vi "Get_Mean_Path_Velocities-1.vi"(4 "error IN":errorcluster, 7 "[IN] Tracks + Starting Position":cluster{"Tracks":dbl[], "Start Pos":i32}[](array[cluster])) -> (0 "error OUT":errorcluster, 3 "[OUT] Mean Path Velocities":dbl[](array[numeric]))   [LabVIEW 2013]
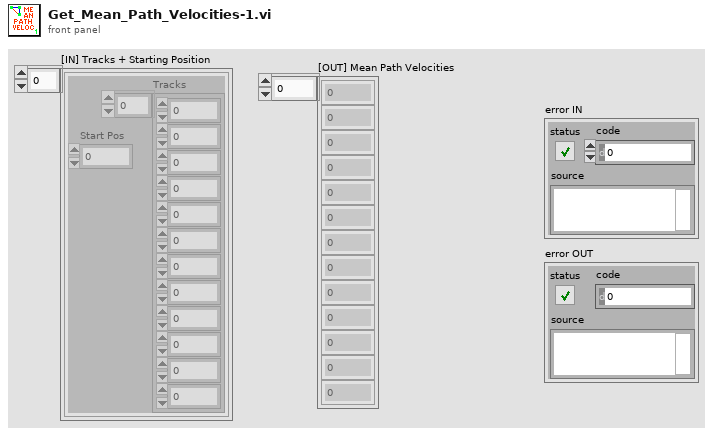
[diagram p1: front panel]
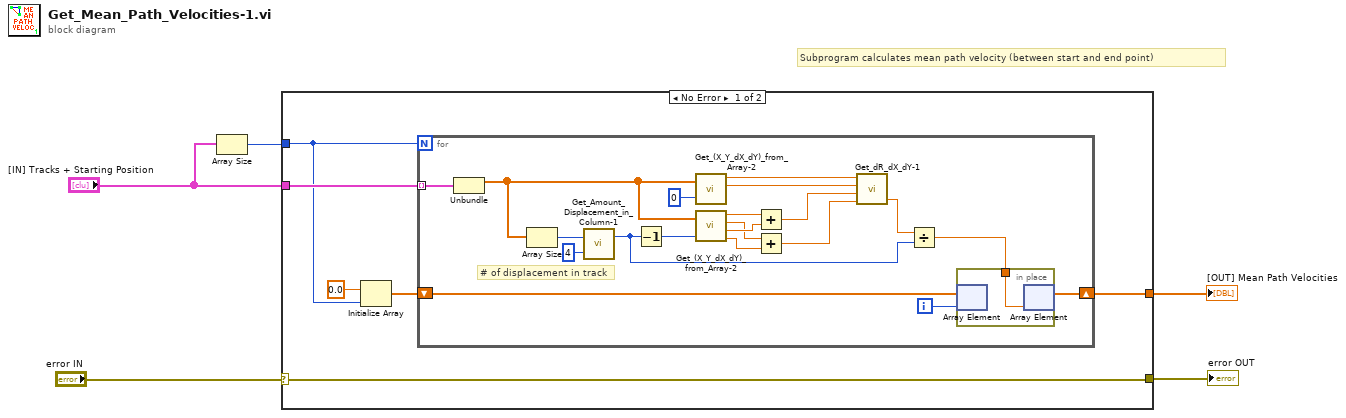
[diagram p0: block diagram]
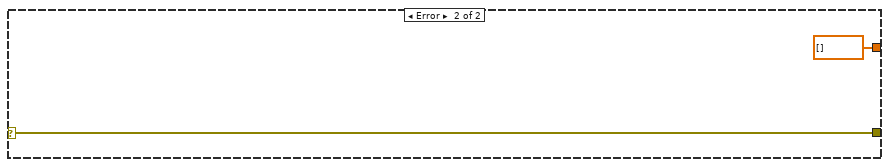
[diagram p2: hidden frame]
diagram:
  # "Subprogram calculates mean path velocity (between start and end point)"
  n1 = Array Size(array="[IN] Tracks + Starting Position") -> (size(s)=w4:i32)
  n2 = case shown="No Error" "error IN" {
    selector: "error IN" -> [w7 w33]
    tunnel: w4 -> [w10 _]
    tunnel: "[IN] Tracks + Starting Position" -> [w11 _]
    tunnel: [w7 w33] -> w2
    tunnel: [w6 dbl[] []] -> w1
    frame No Error {
      n3 = Initialize Array(0.0 ("element"), w10) -> (w8:dbl[])
      n4 = for {
        N: w10 -> [_]
        tunnel: w11 -> [w31] mode=indexing
        shift-right: [w12] -> w6
        shift-left: w8 -> [w15]
        i -> [w14]
        # "# of displacement in track"
        n5 = Unbundle(w31) -> ("Tracks"=w27:dbl[])  [unwired: 1 out]
        n6 = Array Size(array=w27) -> (size(s)=w30:i32)
        n7 = call "Get_Amount_Displacement_in_Column-1.vi"("multiplier"=4, "# Rows"=w30) -> ("Displ amount"=w16:i32)  [unwired: 1 out]
        n8 = Decrement(x=w16) -> (x-1=w26:i32)
        n9 = call "Get_(X_Y_dX_dY)_from_Array-2.vi"("(X,Y,dX,dY)"=w27, "Index of Displacement"=0) -> ("X"=w21:dbl, "Y"=w19:dbl)  [unwired: 2 out]
        n10 = call "Get_(X_Y_dX_dY)_from_Array-2.vi"("(X,Y,dX,dY)"=w27, "Index of Displacement"=w26) -> ("X"=w25:dbl, "Y"=w23:dbl, "dX"=w24:dbl, "dY"=w22:dbl)
        n11 = Add(x=w25, y=w24) -> (x+y=w20:dbl)
        n12 = Add(x=w23, y=w22) -> (x+y=w18:dbl)
        n13 = call "Get_dR_dX_dY-1.vi"("Y2"=w18, "X2"=w20, "Y1"=w19, "X1"=w21) -> ("dR"=w17:dbl)  [unwired: 2 out]
        n14 = Divide(x=w17, y=w16) -> (x/y=w13:dbl)
        n15 = in-place {
          in-place-border: w13 -> [w32]
          n16 = in-place-array #1(w15, w14) -> ()  [unwired: 1 out]
          n17 = in-place-array #1(w32) -> (w12:dbl[])  [unwired: 1 out]
        }
      }
    }
    frame Error {
    }
  }
  "error OUT" <- w2
  "[OUT] Mean Path Velocities" <- w1
